vi "Get - Time Data OBJ.vi"(0 "reference in":refnum<class "HeadAcousticHDF.lvclass">, 5 "error in (no error)":errorcluster) -> (14 "reference out":refnum<class "HeadAcousticHDF.lvclass">, 16 "Time Data OBJ":refnum<class "GSwFormDSP.lvclass">, 19 "error out":errorcluster)   [LabVIEW 2022 SP3, in "HeadAcousticHDF.lvclass"]
uses:
  HeadAcousticHDF.lvclass
  API/GSwFormDSP_class/GSwFormDSP.lvclass
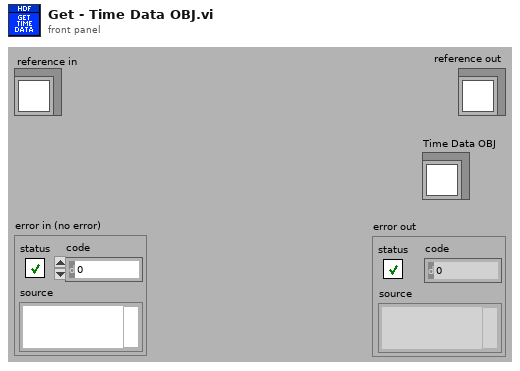
[diagram p1: front panel]
types:
  T1 = typedef "HeadAcousticHDF.lvclass/ObjectAttributes.ctl" = cluster{"Time Data":refnum<class "GSwFormDSP.lvclass">, "Data Plugin Name":string, "Additional Data Plugin Name":string, "New Time Data Obj?":bool}
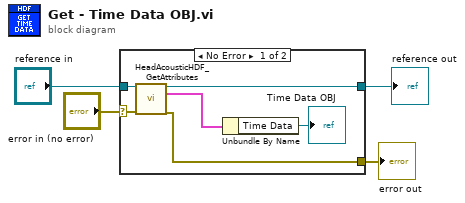
[diagram p0: block diagram]
diagram:
  n1 = case shown="No Error" "error in (no error)" {
    selector: "error in (no error)" -> [w10 w12]
    tunnel: [w9 w12] -> w3
    tunnel: [w8 w11] -> w1
    tunnel: "reference in" -> [w6 w11]
    frame No Error {
      n2 = call "HeadAcousticHDF_GetAttributes.vi"("reference in"=w6, "error in (no error)"=w10) -> ("reference out"=w8:refnum<class "HeadAcousticHDF.lvclass">, "attributes"=w7:T1, "error out"=w9:errorcluster)  [unwired: 14 in, 1 out]
      n3 = Unbundle By Name(w7) -> ("Time Data"=→"Time Data OBJ":refnum<class "GSwFormDSP.lvclass">)
    }
    frame Error {
    }
  }
  "error out" <- w3
  "reference out" <- w1
